vi "Lift State Machine.vi"(8 "Lift Motors B":T1={"DeviceStatus"={"status"=FALSE, "code"=0, "source"=""}, "Type"=enum."PWM", "PWM"={"PWM Channel"=enum."Invalid", "DeadBand"={"Name"="", "maxPositivePwm"=0, "minPositivePwm"=0, "centerPwm"=0, "maxNegativePwm"=0, "minNegativePwm"=0, "angularRange"=0}}, "CAN"={"Device Number"=0, "SetOutput VI Ref"=variant(refnum<vi> refnum), "GetOutput VI Ref"=variant(refnum<vi> refnum), "Enable VI Ref"=variant(refnum<vi> refnum), "Disable VI Ref"=variant(refnum<vi> refnum), "Data"=variant}, "Invert"=FALSE, "DIO PWM"={"PWM \"Enable\" Channel"=enum."Invalid", "DIOChannel"=enum."Invalid", "PWM Rate"=0.0}}, 9 "Lift Motors":T1={"DeviceStatus"={"status"=FALSE, "code"=0, "source"=""}, "Type"=enum."PWM", "PWM"={"PWM Channel"=enum."Invalid", "DeadBand"={"Name"="", "maxPositivePwm"=0, "minPositivePwm"=0, "centerPwm"=0, "maxNegativePwm"=0, "minNegativePwm"=0, "angularRange"=0}}, "CAN"={"Device Number"=0, "SetOutput VI Ref"=variant(enum8{"Percent VBus", "Current", "Speed", "Position", "Voltage"} enum."Percent VBus"), "GetOutput VI Ref"=variant(refnum<k1> refnum), "Enable VI Ref"=variant(dbl 12.0), "Disable VI Ref"=variant(enum8{"Percent VBus", "Speed", "Position", "Slave", "Unchanged / Invalid"} enum."Percent VBus"), "Data"=variant}, "Invert"=FALSE, "DIO PWM"={"PWM \"Enable\" Channel"=enum."Invalid", "DIOChannel"=enum."Invalid", "PWM Rate"=0.0}}) -> ()   [LabVIEW 2017]
uses:
  <vilib>/Rock Robotics/WPI/MotorControl/WPI_MotorControlDeviceRef.ctl
  <vilib>/Rock Robotics/WPI/MotorControl/WPI_MotorControlType.ctl
  <vilib>/Rock Robotics/SystemInterfaces/DIO/FPGA_DIOPWMChannel.ctl
  <vilib>/Rock Robotics/WPI/PWM/WPI_PWMDeadband.ctl
  <vilib>/Rock Robotics/SystemInterfaces/DIO/FPGA_DIOChannel.ctl
  Lift States.ctl
  Robot Global Data.vi
panel:
  in  "Rock Bottom Down Speed":dbl=-0.1
  in  "Almost Down Setpoint":dbl=0.1
  in  "Soft Limits?":bool=TRUE
  in  "Lift Max Position":dbl=0.98
  in  "Lift Min Position":dbl
  in  "Max Lift Speed":dbl=1.0
  in  "Min Lift Speed":dbl=0.5
  in  "Kp":dbl=5.0
  in  "Scale High Setpoint":dbl=0.94
  in  "Scale Med Setpoint":dbl=0.6
  in  "Scale Low Setpoint":dbl=0.35
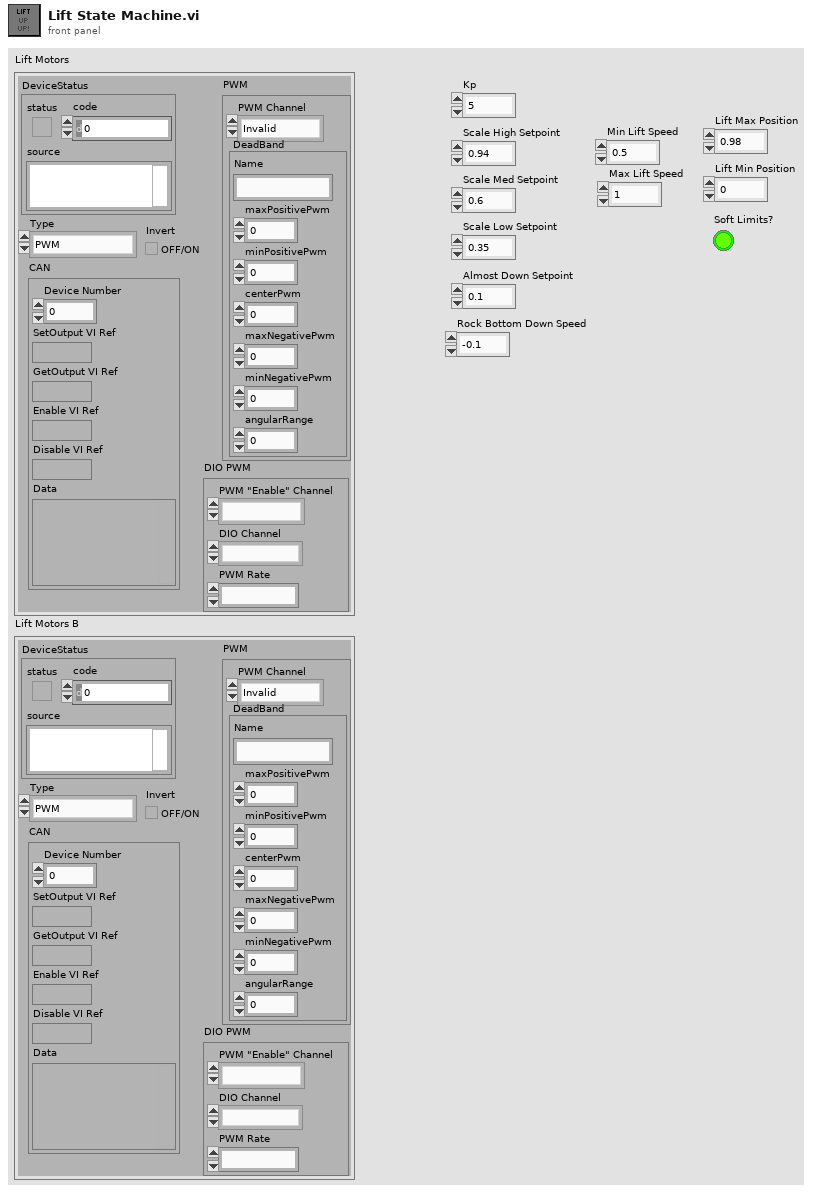
[diagram p1: front panel]
types:
  T1 = typedef "WPI_MotorControlDeviceRef.ctl" = cluster{"DeviceStatus":errorcluster, "Type":T2, "PWM":cluster{"PWM Channel":T3, "DeadBand":T4}, "CAN":cluster{"Device Number":u8, "SetOutput VI Ref":variant, "GetOutput VI Ref":variant, "Enable VI Ref":variant, "Disable VI Ref":variant, "Data":variant}, "Invert":bool, "DIO PWM":cluster{"PWM \"Enable\" Channel":T3, "DIOChannel":T5, "PWM Rate":dbl}}
  T2 = typedef "WPI_MotorControlType.ctl" = enum16{"PWM", "CAN", "DIO PWM"}
  T3 = typedef "FPGA_DIOPWMChannel.ctl" = enum8{"PWM 0", "PWM 1", "PWM 2", "PWM 3", "PWM 4", "PWM 5", "PWM 6", "PWM 7", "PWM 8", "PWM 9", "PWM MXP 0", "PWM MXP 1", "PWM MXP 2", "PWM MXP 3", "PWM MXP 4", "PWM MXP 5", "PWM MXP 6", "PWM MXP 7", "PWM MXP 8", "PWM MXP 9", "Invalid"}
  T4 = typedef "WPI_PWMDeadband.ctl" = cluster{"Name":string, "maxPositivePwm":i32, "minPositivePwm":i32, "centerPwm":i32, "maxNegativePwm":i32, "minNegativePwm":i32, "angularRange":u16}
  T5 = typedef "FPGA_DIOChannel.ctl" = enum8{"DIO 0", "DIO 1", "DIO 2", "DIO 3", "DIO 4", "DIO 5", "DIO 6", "DIO 7", "DIO 8", "DIO 9", "DIO MXP 0", "DIO MXP 1", "DIO MXP 2", "DIO MXP 3", "DIO MXP 4", "DIO MXP 5", "DIO MXP 6", "DIO MXP 7", "DIO MXP 8", "DIO MXP 9", "DIO MXP 10", "DIO MXP 11", "DIO MXP 12", "DIO MXP 13", "DIO MXP 14", "DIO MXP 15", "SPI Port CS1", "SPI Port CS2", "SPI Port CS3", "SPI Port MISO", "SPI Port MOSI", "Invalid"}
  T6 = typedef "Lift States.ctl" = enum16{"Manual", "Scale Low", "Scale Middle", "Scale High", "Rock Bottom", "Almost Down"}
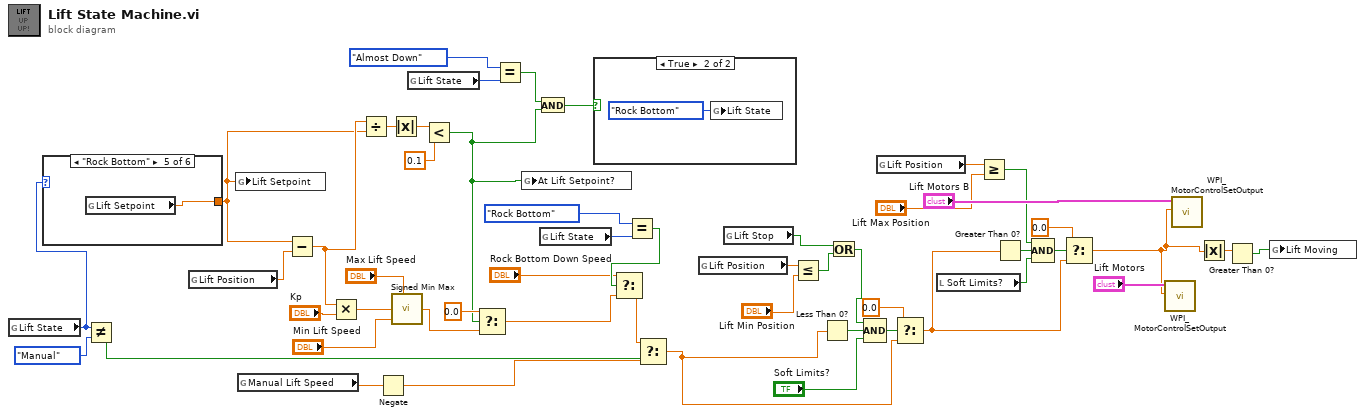
[diagram p0: block diagram]
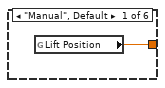
[diagram p3: hidden frame]
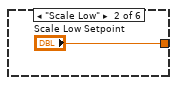
[diagram p4: hidden frame]
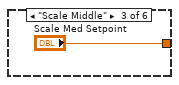
[diagram p5: hidden frame]
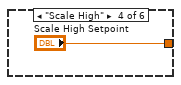
[diagram p6: hidden frame]
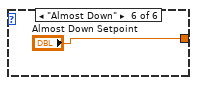
[diagram p7: hidden frame]
diagram:
  n1 = global read "Robot Global Data.vi" "Lift State"() -> (w47:T6)
  n2 = case shown="\"Rock Bottom\"" w47 {
    tunnel: [w52 "Scale Low Setpoint" "Scale Med Setpoint" "Scale High Setpoint" w56 "Almost Down Setpoint"] -> w43
    frame "Manual", Default {
      n3 = global read "Robot Global Data.vi" "Lift Position"() -> (w52:dbl)
    }
    frame "Scale Low" {
    }
    frame "Scale Middle" {
    }
    frame "Scale High" {
    }
    frame "Rock Bottom" {
      n4 = global read "Robot Global Data.vi" "Lift Setpoint"() -> (w56:dbl)
    }
    frame "Almost Down" {
    }
  }
  n5 = Not Equal?(x=w47, y=Lift_States."Manual") -> (x != y?=w45:bool)
  n6 = global read "Robot Global Data.vi" "Lift Position"() -> (w48:dbl)
  n7 = global write "Robot Global Data.vi" "Lift Setpoint"(w43) -> ()
  n8 = global read "Robot Global Data.vi" "Manual Lift Speed"() -> (w38:dbl)
  n9 = Subtract(x=w43, y=w48) -> (x-y=w44:dbl)
  n10 = Multiply(x=w44, y="Kp") -> (x*y=w41:dbl)
  n11 = Divide(x=w44, y=w43) -> (x/y=w17:dbl)
  n12 = Negate(x=w38) -> (-x=w37:dbl)
  n13 = Absolute Value(x=w17) -> (abs(x)=w18:dbl)
  n14 = call "Signed Min Max.vi"("Min"="Min Lift Speed", "Value"=w41, "Max"="Max Lift Speed") -> ("Output"=w16:dbl)  [unwired: 2 in]
  n15 = global read "Robot Global Data.vi" "Lift State"() -> (w14:T6)
  n16 = Less?(x=w18, y=0.1) -> (x < y?=w1:bool)
  n17 = Select(t=0.0, s=w1, f=w16) -> (s? t:f=w7:dbl)
  n18 = Equal?(x=Lift_States."Almost Down", y=w14) -> (x = y?=w12:bool)
  n19 = global write "Robot Global Data.vi" "At Lift Setpoint?"(w1) -> ()
  n20 = And(x=w12, y=w1) -> (x .and. y?=w11:bool)
  n21 = global read "Robot Global Data.vi" "Lift State"() -> (w10:T6)
  n22 = case shown="True" w11 {
    frame False {
    }
    frame True {
      n23 = global write "Robot Global Data.vi" "Lift State"(Lift_States."Rock Bottom" ("Lift State")) -> ()
    }
  }
  n24 = Equal?(x=Lift_States."Rock Bottom", y=w10) -> (x = y?=w8:bool)
  n25 = Select(t="Rock Bottom Down Speed", s=w8, f=w7) -> (s? t:f=w6:dbl)
  n26 = Select(t=w6, s=w45, f=w37) -> (s? t:f=w23:dbl)
  n27 = global read "Robot Global Data.vi" "Lift Position"() -> (w36:dbl)
  n28 = global read "Robot Global Data.vi" "Lift Stop"() -> (w19:bool)
  n29 = Less Or Equal?(x=w36, y="Lift Min Position") -> (x <= y?=w21:bool)
  n30 = Less Than 0?(x=w23) -> (x < 0?=w34:bool)
  n31 = Or(x=w19, y=w21) -> (x .or. y?=w20:bool)
  n32 = Compound Arithmetic op=AND(w20, w34, "Soft Limits?") -> (w35:bool)
  n33 = global read "Robot Global Data.vi" "Lift Position"() -> (w32:dbl)
  n34 = Select(t=0.0, s=w35, f=w23) -> (s? t:f=w22:dbl)
  n35 = local read "Soft Limits?"() -> (w26:bool)
  n36 = Greater Or Equal?(x=w32, y="Lift Max Position") -> (x >= y?=w29:bool)
  n37 = Greater Than 0?(x=w22) -> (x > 0?=w28:bool)
  n38 = Compound Arithmetic op=AND(w29, w28, w26) -> (w30:bool)
  n39 = Select(t=0.0, s=w30, f=w22) -> (s? t:f=w4:dbl)
  n40 = call <vilib>:"WPI_MotorControlSetOutput.vi"("Output"=w4, "MotorControlDevRef"="Lift Motors") -> ()  [unwired: 7 in, 3 out]
  n41 = call <vilib>:"WPI_MotorControlSetOutput.vi"("Output"=w4, "MotorControlDevRef"="Lift Motors B") -> ()  [unwired: 7 in, 3 out]
  n42 = Absolute Value(x=w4) -> (abs(x)=w3:dbl)
  n43 = Greater Than 0?(x=w3) -> (x > 0?=w2:bool)
  n44 = global write "Robot Global Data.vi" "Lift Moving"(w2) -> ()
